vi "AutoMapper.vi"(8 "error in (no error)":errorcluster) -> (0 "error out 4":errorcluster={"status"=TRUE, "code"=1055, "source"="Property Node (arg 1) in AutoMapper.vi->Main.vi"})   [LabVIEW 2014]
uses:
  Libraries/Map Data Folder/All-Lines.ctl
  Libraries/Map Data Folder/LineCluster.ctl
  Libraries/Map Data Folder/LineConnection.ctl
  <vilib>/Utility/miscctls.llb/LVCursorListTypeDef.ctl
  <vilib>/Utility/miscctls.llb/LVRangeTypeDef.ctl
  <vilib>/Utility/miscctls.llb/LVPoint32TypeDef.ctl
  Controls/SwitchOp.ctl
  SwitchControl/Controls/ManualOveride.ctl
  SwitchControl/Controls/ManualState.ctl
  Libraries/Map Data Folder/Map Data.lvlib
  Libraries/Contact Data/Contact Data.lvlib
panel:
  in  "SwitchOp":T1[](array[typedef])
  out "Cursor List":T4
  out "output array":T5
  out "AutoMapper":cluster{cluster{"X":dbl, "Z":dbl}[]}[](graph)=[{[{"X"=1846.876, "Z"=5458.5}, {"X"=1845.414, "Z"=5458.5}, {"X"=1843.46, "Z"=5458.5}, {"X"=1841.231, "Z"=5458.5}, {"X"=1838.753, "Z"=5458.5}, {"X"=1836.154, "Z"=5458.5}, {"X"=1833.319, "Z"=5458.5}, {"X"=1830.276, "Z"=5458.5}, {"X"=1827.045, "Z"=5458.5}, {"X"=1823.657, "Z"=5458.5}, {"X"=1820.23, "Z"=5458.5}, {"X"=1816.783, "Z"=5458.5}, {"X"=1813.318, "Z"=5458.5}, {"X"=1809.835, "Z"=5458.5}, {"X"=1806.336, "Z"=5458.5}, {"X"=1802.822, "Z"=5458.5}, {"X"=1799.293, "Z"=5458.5}, {"X"=1795.751, "Z"=5458.5}, {"X"=1792.197, "Z"=5458.5}, {"X"=1788.356, "Z"=5458.5}, {"X"=1784.777, "Z"=5458.5}, {"X"=1782.771, "Z"=5458.749}, {"X"=1781.189, "Z"=5458.5}, {"X"=1777.591, "Z"=5458.5}, {"X"=1775.817, "Z"=5458.5}, {"X"=1773.983, "Z"=5458.5}, {"X"=1772.669, "Z"=5458.5}, {"X"=1770.367, "Z"=5458.5}, {"X"=1769.342, "Z"=5458.5}, {"X"=1766.743, "Z"=5458.5}, {"X"=1763.943, "Z"=5458.5}, {"X"=1762.831, "Z"=5458.5}, {"X"=1759.192, "Z"=5458.5}, {"X"=1755.545, "Z"=5458.5}, {"X"=1751.893, "Z"=5458.5}, {"X"=1749.392, "Z"=5458.5}, {"X"=1748.234, "Z"=5458.5}, {"X"=1744.57, "Z"=5458.5}, {"X"=1743.098, "Z"=5458.5}, {"X"=1740.9, "Z"=5458.5}, {"X"=1737.225, "Z"=5458.5}, {"X"=1735.038, "Z"=5458.5}, {"X"=1733.546, "Z"=5458.5}, {"X"=1729.862, "Z"=5458.5}, {"X"=1726.174, "Z"=5458.5}, {"X"=1722.481, "Z"=5458.5}, {"X"=1718.785, "Z"=5458.507}, {"X"=1714.804, "Z"=5458.598}, {"X"=1711.11, "Z"=5458.842}, {"X"=1707.431, "Z"=5459.274}, {"X"=1703.781, "Z"=5459.918}, {"X"=1700.177, "Z"=5460.798}, {"X"=1696.639, "Z"=5461.934}, {"X"=1693.093, "Z"=5463.377}, {"X"=1689.52, "Z"=5465.176}, {"X"=1685.962, "Z"=5467.324}, {"X"=1682.433, "Z"=5469.784}, {"X"=1678.913, "Z"=5472.481}, {"X"=1675.343, "Z"=5475.315}, {"X"=1671.345, "Z"=5478.377}, {"X"=1667.401, "Z"=5481.085}, {"X"=1663.17, "Z"=5483.523}, {"X"=1658.281, "Z"=5485.722}, {"X"=1653.463, "Z"=5487.302}, {"X"=1648.432, "Z"=5488.426}, {"X"=1643.243, "Z"=5489.125}, {"X"=1637.941, "Z"=5489.446}, {"X"=1632.556, "Z"=5489.5}, {"X"=1627.102, "Z"=5489.5}, {"X"=1621.583, "Z"=5489.5}, {"X"=1615.139, "Z"=5489.5}, {"X"=1609.49, "Z"=5489.5}, {"X"=1603.785, "Z"=5489.5}, {"X"=1598.026, "Z"=5489.5}, {"X"=1591.766, "Z"=5489.5}, {"X"=1585.902, "Z"=5489.5}, {"X"=1579.991, "Z"=5489.5}, {"X"=1573.574, "Z"=5489.5}, {"X"=1567.106, "Z"=5489.5}, {"X"=1561.057, "Z"=5489.5}, {"X"=1554.968, "Z"=5489.5}, {"X"=1548.839, "Z"=5489.5}, {"X"=1542.673, "Z"=5489.5}, {"X"=1536.471, "Z"=5489.5}, {"X"=1530.234, "Z"=5489.5}, {"X"=1523.963, "Z"=5489.5}, {"X"=1517.66, "Z"=5489.5}, {"X"=1511.326, "Z"=5489.5}, {"X"=1504.961, "Z"=5489.5}, {"X"=1498.073, "Z"=5489.5}, {"X"=1491.648, "Z"=5489.5}, {"X"=1485.196, "Z"=5489.5}, {"X"=1478.717, "Z"=5489.5}, {"X"=1472.213, "Z"=5489.5}, {"X"=1465.683, "Z"=5489.502}, {"X"=1458.638, "Z"=5489.822}, {"X"=1452.145, "Z"=5490.832}, {"X"=1445.783, "Z"=5492.571}, {"X"=1439.639, "Z"=5495.023}, {"X"=1433.355, "Z"=5498.431}, {"X"=1427.912, "Z"=5502.268}, {"X"=1422.92, "Z"=5506.705}, {"X"=1418.125, "Z"=5512.094}, {"X"=1414.278, "Z"=5517.602}, {"X"=1411.074, "Z"=5523.528}, {"X"=1408.565, "Z"=5529.8}, {"X"=1406.792, "Z"=5536.335}, {"X"=1405.782, "Z"=5543.048}, {"X"=1405.501, "Z"=5549.849}, {"X"=1405.5, "Z"=5556.676}, {"X"=1405.5, "Z"=5563.519}, {"X"=1405.5, "Z"=5570.376}, {"X"=1405.5, "Z"=5577.248}, {"X"=1405.5, "Z"=5584.126}, {"X"=1405.5, "Z"=5590.852}, {"X"=1405.5, "Z"=5597.365}, {"X"=1405.5, "Z"=5604.141}, {"X"=1405.5, "Z"=5610.209}, {"X"=1405.5, "Z"=5616.063}, {"X"=1405.5, "Z"=5621.699}, {"X"=1405.5, "Z"=5627.118}, {"X"=1405.5, "Z"=5631.758}, {"X"=1405.5, "Z"=5634.602}]}, {[{"X"=1401.5, "Z"=5594.986}, {"X"=1401.5, "Z"=5593.692}, {"X"=1401.5, "Z"=5586.908}, {"X"=1401.5, "Z"=5585.809}, {"X"=1401.5, "Z"=5584.365}, {"X"=1401.5, "Z"=5582.58}, {"X"=1401.5, "Z"=5580.516}, {"X"=1401.5, "Z"=5578.212}, {"X"=1401.5, "Z"=5575.693}, {"X"=1401.5, "Z"=5572.979}, {"X"=1401.5, "Z"=5570.085}, {"X"=1401.5, "Z"=5567.024}, {"X"=1401.5, "Z"=5563.807}, {"X"=1401.5, "Z"=5560.442}, {"X"=1401.5, "Z"=5556.938}, {"X"=1401.5, "Z"=5553.299}, {"X"=1401.5, "Z"=5549.534}, {"X"=1401.502, "Z"=5545.646}, {"X"=1401.6, "Z"=5541.644}, {"X"=1401.939, "Z"=5537.543}, {"X"=1402.583, "Z"=5533.368}, {"X"=1403.554, "Z"=5529.149}, {"X"=1404.983, "Z"=5524.592}, {"X"=1406.681, "Z"=5520.384}, {"X"=1408.745, "Z"=5516.235}, {"X"=1411.382, "Z"=5511.877}, {"X"=1414.218, "Z"=5507.974}, {"X"=1417.682, "Z"=5503.971}, {"X"=1421.274, "Z"=5500.485}, {"X"=1425.214, "Z"=5497.263}, {"X"=1429.827, "Z"=5494.138}, {"X"=1434.432, "Z"=5491.6}, {"X"=1439.704, "Z"=5489.309}, {"X"=1444.857, "Z"=5487.633}, {"X"=1450.636, "Z"=5486.355}, {"X"=1457.03, "Z"=5485.632}, {"X"=1462.687, "Z"=5485.499}, {"X"=1468.863, "Z"=5485.5}, {"X"=1474.669, "Z"=5485.5}, {"X"=1480.997, "Z"=5485.5}, {"X"=1486.943, "Z"=5485.5}, {"X"=1492.955, "Z"=5485.5}, {"X"=1499.501, "Z"=5485.5}, {"X"=1505.645, "Z"=5485.5}, {"X"=1512.332, "Z"=5485.5}, {"X"=1518.605, "Z"=5485.5}, {"X"=1524.939, "Z"=5485.5}, {"X"=1531.332, "Z"=5485.5}, {"X"=1537.784, "Z"=5485.5}, {"X"=1544.796, "Z"=5485.5}, {"X"=1551.367, "Z"=5485.5}, {"X"=1557.995, "Z"=5485.5}, {"X"=1564.677, "Z"=5485.5}, {"X"=1571.415, "Z"=5485.5}, {"X"=1578.206, "Z"=5485.5}, {"X"=1585.051, "Z"=5485.5}, {"X"=1591.948, "Z"=5485.5}, {"X"=1599.434, "Z"=5485.5}, {"X"=1606.438, "Z"=5485.5}, {"X"=1613.494, "Z"=5485.5}, {"X"=1620.599, "Z"=5485.5}, {"X"=1627.753, "Z"=5485.5}, {"X"=1634.956, "Z"=5485.444}, {"X"=1642.182, "Z"=5484.911}, {"X"=1649.898, "Z"=5483.451}, {"X"=1656.845, "Z"=5481.087}, {"X"=1663.408, "Z"=5477.702}, {"X"=1669.536, "Z"=5473.49}, {"X"=1675.426, "Z"=5468.866}, {"X"=1680.506, "Z"=5465.006}, {"X"=1681.928, "Z"=5464.014}, {"X"=1683.425, "Z"=5463.025}, {"X"=1685.221, "Z"=5461.92}, {"X"=1686.784, "Z"=5461.032}, {"X"=1688.448, "Z"=5460.162}, {"X"=1689.514, "Z"=5459.645}, {"X"=1692.148, "Z"=5458.502}, {"X"=1694.602, "Z"=5457.596}, {"X"=1696.064, "Z"=5457.125}, {"X"=1697.726, "Z"=5456.647}, {"X"=1700.823, "Z"=5455.909}, {"X"=1703.533, "Z"=5455.412}, {"X"=1707.824, "Z"=5454.868}, {"X"=1711.202, "Z"=5454.627}, {"X"=1715.302, "Z"=5454.512}, {"X"=1718.959, "Z"=5454.5}, {"X"=1722.952, "Z"=5454.5}, {"X"=1726.761, "Z"=5454.5}, {"X"=1728.143, "Z"=5454.5}, {"X"=1729.73, "Z"=5454.5}, {"X"=1730.767, "Z"=5454.5}, {"X"=1734.605, "Z"=5454.5}, {"X"=1743.09, "Z"=5454.5}, {"X"=1744.603, "Z"=5454.5}, {"X"=1746.155, "Z"=5454.5}, {"X"=1747.277, "Z"=5454.5}, {"X"=1748.888, "Z"=5454.5}, {"X"=1750.944, "Z"=5454.5}, {"X"=1752.514, "Z"=5454.5}, {"X"=1754.254, "Z"=5454.5}, {"X"=1755.425, "Z"=5454.5}, {"X"=1756.626, "Z"=5454.5}, {"X"=1758.764, "Z"=5454.5}, {"X"=1760.384, "Z"=5454.5}, {"X"=1761.686, "Z"=5454.5}, {"X"=1763.01, "Z"=5454.5}, {"X"=1765.01, "Z"=5454.5}, {"X"=1766.549, "Z"=5454.5}, {"X"=1768.513, "Z"=5454.5}, {"X"=1769.936, "Z"=5454.5}, {"X"=1771.064, "Z"=5454.5}, {"X"=1772.836, "Z"=5454.5}, {"X"=1774.09, "Z"=5454.5}, {"X"=1775.959, "Z"=5454.5}, {"X"=1777.402, "Z"=5454.5}, {"X"=1779.54, "Z"=5454.5}, {"X"=1781.08, "Z"=5454.5}, {"X"=1783.115, "Z"=5454.5}, {"X"=1786.384, "Z"=5454.5}, {"X"=1788.654, "Z"=5454.5}, {"X"=1791.126, "Z"=5454.5}, {"X"=1794.012, "Z"=5454.5}, {"X"=1795.833, "Z"=5454.5}, {"X"=1799.183, "Z"=5454.5}, {"X"=1800.864, "Z"=5454.5}, {"X"=1804.158, "Z"=5454.5}, {"X"=1805.5, "Z"=5454.5}, {"X"=1808.926, "Z"=5454.5}, {"X"=1810.101, "Z"=5454.5}, {"X"=1813.478, "Z"=5454.5}, {"X"=1814.667, "Z"=5454.5}, {"X"=1817.8, "Z"=5454.5}, {"X"=1819.199, "Z"=5454.5}, {"X"=1821.878, "Z"=5454.5}, {"X"=1823.697, "Z"=5454.5}, {"X"=1825.693, "Z"=5454.5}, {"X"=1828.16, "Z"=5454.5}, {"X"=1829.224, "Z"=5454.5}, {"X"=1832.575, "Z"=5454.5}, {"X"=1835.51, "Z"=5454.5}, {"X"=1837.151, "Z"=5454.5}, {"X"=1840.345, "Z"=5454.5}]}, {[{"X"=1799.071, "Z"=5459.117}, {"X"=1801.212, "Z"=5460.627}, {"X"=1803.251, "Z"=5462.366}, {"X"=1805.161, "Z"=5464.328}, {"X"=1807.039, "Z"=5466.683}, {"X"=1808.583, "Z"=5469.081}, {"X"=1809.905, "Z"=5471.669}, {"X"=1810.976, "Z"=5474.425}, {"X"=1811.769, "Z"=5477.325}, {"X"=1812.261, "Z"=5480.341}, {"X"=1812.464, "Z"=5483.437}, {"X"=1812.5, "Z"=5486.593}, {"X"=1812.5, "Z"=5489.795}, {"X"=1812.5, "Z"=5493.04}, {"X"=1812.5, "Z"=5496.583}, {"X"=1812.5, "Z"=5499.916}, {"X"=1812.5, "Z"=5503.29}, {"X"=1812.5, "Z"=5506.969}, {"X"=1812.5, "Z"=5509.183}, {"X"=1812.5, "Z"=5510.425}, {"X"=1812.5, "Z"=5513.919}, {"X"=1812.5, "Z"=5517.45}, {"X"=1812.5, "Z"=5521.018}, {"X"=1812.5, "Z"=5524.901}, {"X"=1812.5, "Z"=5528.543}, {"X"=1812.5, "Z"=5530.174}, {"X"=1812.5, "Z"=5532.504}, {"X"=1812.5, "Z"=5536.217}, {"X"=1812.5, "Z"=5539.963}, {"X"=1812.5, "Z"=5544.034}, {"X"=1812.5, "Z"=5547.847}, {"X"=1812.5, "Z"=5551.692}, {"X"=1812.5, "Z"=5555.692}, {"X"=1812.5, "Z"=5559.942}, {"X"=1812.5, "Z"=5564.425}, {"X"=1812.5, "Z"=5569.129}, {"X"=1812.5, "Z"=5574.042}, {"X"=1812.5, "Z"=5579.155}, {"X"=1812.5, "Z"=5584.457}, {"X"=1812.5, "Z"=5589.942}, {"X"=1812.5, "Z"=5595.603}, {"X"=1812.5, "Z"=5601.432}, {"X"=1812.5, "Z"=5607.425}, {"X"=1812.5, "Z"=5613.577}, {"X"=1812.5, "Z"=5617.536}, {"X"=1812.5, "Z"=5619.882}, {"X"=1812.5, "Z"=5626.335}, {"X"=1812.5, "Z"=5633.447}, {"X"=1812.5, "Z"=5639.076}, {"X"=1812.5, "Z"=5640.722}, {"X"=1812.5, "Z"=5647.62}, {"X"=1812.5, "Z"=5654.65}, {"X"=1812.5, "Z"=5660.65}, {"X"=1812.5, "Z"=5661.812}, {"X"=1812.5, "Z"=5669.666}, {"X"=1812.5, "Z"=5677.089}, {"X"=1812.5, "Z"=5682.259}, {"X"=1812.5, "Z"=5684.634}, {"X"=1812.5, "Z"=5692.297}, {"X"=1812.5, "Z"=5700.065}, {"X"=1812.5, "Z"=5703.903}, {"X"=1812.5, "Z"=5707.786}, {"X"=1812.5, "Z"=5715.309}, {"X"=1812.5, "Z"=5722.623}, {"X"=1812.5, "Z"=5725.581}, {"X"=1812.5, "Z"=5729.728}, {"X"=1812.5, "Z"=5736.621}, {"X"=1812.5, "Z"=5743.341}, {"X"=1812.5, "Z"=5747.281}, {"X"=1812.5, "Z"=5750.016}, {"X"=1812.5, "Z"=5756.657}, {"X"=1812.474, "Z"=5763.262}, {"X"=1812.185, "Z"=5769.825}, {"X"=1811.458, "Z"=5776.319}, {"X"=1810.766, "Z"=5782.782}, {"X"=1810.518, "Z"=5789.243}, {"X"=1810.506, "Z"=5790.562}, {"X"=1810.5, "Z"=5795.676}, {"X"=1810.5, "Z"=5802.074}, {"X"=1810.5, "Z"=5808.438}, {"X"=1810.5, "Z"=5812.263}, {"X"=1810.5, "Z"=5814.768}, {"X"=1810.5, "Z"=5821.063}, {"X"=1810.5, "Z"=5827.804}, {"X"=1810.5, "Z"=5834.027}, {"X"=1810.5, "Z"=5835.615}, {"X"=1810.498, "Z"=5840.216}, {"X"=1810.209, "Z"=5846.832}, {"X"=1809.284, "Z"=5852.872}, {"X"=1808.217, "Z"=5857.088}, {"X"=1807.703, "Z"=5858.738}, {"X"=1805.493, "Z"=5864.361}, {"X"=1802.455, "Z"=5870.07}, {"X"=1799.074, "Z"=5874.99}, {"X"=1798.165, "Z"=5876.137}, {"X"=1795.206, "Z"=5879.491}, {"X"=1790.905, "Z"=5883.531}, {"X"=1786.226, "Z"=5887.07}, {"X"=1780.833, "Z"=5890.283}, {"X"=1775.559, "Z"=5892.685}, {"X"=1770.093, "Z"=5894.503}, {"X"=1764.5, "Z"=5895.731}, {"X"=1760.983, "Z"=5896.193}, {"X"=1758.844, "Z"=5896.365}, {"X"=1753.186, "Z"=5896.5}, {"X"=1747.553, "Z"=5896.5}, {"X"=1741.942, "Z"=5896.5}, {"X"=1739.313, "Z"=5896.5}, {"X"=1736.351, "Z"=5896.5}, {"X"=1730.782, "Z"=5896.5}, {"X"=1725.234, "Z"=5896.5}, {"X"=1719.705, "Z"=5896.5}, {"X"=1717.619, "Z"=5896.5}, {"X"=1714.169, "Z"=5896.5}, {"X"=1708.622, "Z"=5896.5}, {"X"=1703.065, "Z"=5896.5}, {"X"=1697.496, "Z"=5896.5}, {"X"=1695.925, "Z"=5896.5}, {"X"=1691.917, "Z"=5896.5}, {"X"=1686.327, "Z"=5896.5}, {"X"=1680.726, "Z"=5896.5}, {"X"=1675.115, "Z"=5896.5}, {"X"=1672.569, "Z"=5896.5}, {"X"=1669.494, "Z"=5896.5}, {"X"=1663.862, "Z"=5896.5}, {"X"=1658.219, "Z"=5896.5}, {"X"=1652.567, "Z"=5896.5}, {"X"=1650.865, "Z"=5896.5}, {"X"=1646.905, "Z"=5896.5}, {"X"=1641.232, "Z"=5896.5}, {"X"=1635.55, "Z"=5896.5}, {"X"=1629.857, "Z"=5896.5}, {"X"=1624.155, "Z"=5896.5}, {"X"=1618.443, "Z"=5896.5}, {"X"=1612.723, "Z"=5896.431}, {"X"=1607.023, "Z"=5895.916}, {"X"=1601.407, "Z"=5894.762}, {"X"=1595.949, "Z"=5892.975}, {"X"=1590.721, "Z"=5890.578}, {"X"=1587.306, "Z"=5888.597}, {"X"=1585.788, "Z"=5887.6}, {"X"=1581.215, "Z"=5884.081}, {"X"=1577.061, "Z"=5880.062}, {"X"=1573.379, "Z"=5875.595}, {"X"=1571.948, "Z"=5873.537}, {"X"=1570.222, "Z"=5870.733}, {"X"=1567.633, "Z"=5865.535}, {"X"=1565.653, "Z"=5860.067}, {"X"=1564.313, "Z"=5854.399}, {"X"=1563.604, "Z"=5848.158}, {"X"=1563.5, "Z"=5842.311}, {"X"=1563.5, "Z"=5836.453}, {"X"=1563.5, "Z"=5831.83}, {"X"=1563.503, "Z"=5830.586}, {"X"=1563.759, "Z"=5824.72}, {"X"=1564.64, "Z"=5818.91}, {"X"=1566.193, "Z"=5813.234}, {"X"=1567.159, "Z"=5810.611}, {"X"=1568.396, "Z"=5807.769}, {"X"=1571.222, "Z"=5802.589}, {"X"=1574.634, "Z"=5797.764}, {"X"=1578.584, "Z"=5793.357}, {"X"=1583.02, "Z"=5789.43}, {"X"=1587.888, "Z"=5786.037}, {"X"=1593.125, "Z"=5783.229}, {"X"=1597.481, "Z"=5781.454}, {"X"=1598.66, "Z"=5781.05}, {"X"=1604.421, "Z"=5779.535}, {"X"=1610.328, "Z"=5778.705}, {"X"=1616.762, "Z"=5778.499}, {"X"=1618.836, "Z"=5778.5}, {"X"=1622.75, "Z"=5778.5}, {"X"=1628.747, "Z"=5778.5}, {"X"=1635.212, "Z"=5778.5}, {"X"=1641.224, "Z"=5778.5}, {"X"=1647.244, "Z"=5778.5}, {"X"=1653.27, "Z"=5778.5}, {"X"=1659.304, "Z"=5778.5}, {"X"=1662.216, "Z"=5778.5}, {"X"=1665.346, "Z"=5778.5}, {"X"=1671.394, "Z"=5778.5}, {"X"=1677.45, "Z"=5778.5}, {"X"=1683.513, "Z"=5778.5}, {"X"=1689.583, "Z"=5778.5}, {"X"=1695.66, "Z"=5778.5}, {"X"=1701.744, "Z"=5778.5}, {"X"=1705.597, "Z"=5778.5}, {"X"=1707.835, "Z"=5778.5}, {"X"=1713.932, "Z"=5778.533}, {"X"=1720.03, "Z"=5778.8}, {"X"=1726.102, "Z"=5779.467}, {"X"=1728.88, "Z"=5779.922}, {"X"=1732.127, "Z"=5780.524}, {"X"=1738.16, "Z"=5781.57}, {"X"=1744.255, "Z"=5782.219}, {"X"=1750.386, "Z"=5782.471}, {"X"=1756.53, "Z"=5782.458}, {"X"=1762.675, "Z"=5782.2}, {"X"=1768.804, "Z"=5781.616}, {"X"=1771.5, "Z"=5781.231}, {"X"=1774.883, "Z"=5780.617}, {"X"=1781.307, "Z"=5778.941}, {"X"=1787.045, "Z"=5776.677}, {"X"=1792.387, "Z"=5773.591}, {"X"=1797.105, "Z"=5769.613}, {"X"=1800.993, "Z"=5764.814}, {"X"=1803.959, "Z"=5759.385}, {"X"=1806.054, "Z"=5753.552}, {"X"=1807.41, "Z"=5747.494}, {"X"=1808.212, "Z"=5740.847}, {"X"=1808.478, "Z"=5734.627}, {"X"=1808.5, "Z"=5728.394}, {"X"=1808.5, "Z"=5722.154}, {"X"=1808.5, "Z"=5715.908}, {"X"=1808.5, "Z"=5709.657}, {"X"=1808.5, "Z"=5703.4}, {"X"=1808.5, "Z"=5702.389}, {"X"=1808.5, "Z"=5697.137}, {"X"=1808.5, "Z"=5695.208}, {"X"=1808.5, "Z"=5688.938}, {"X"=1808.5, "Z"=5684.571}, {"X"=1808.5, "Z"=5682.661}, {"X"=1808.5, "Z"=5676.379}, {"X"=1808.5, "Z"=5670.091}, {"X"=1808.5, "Z"=5667.105}, {"X"=1808.5, "Z"=5663.798}, {"X"=1808.5, "Z"=5657.499}, {"X"=1808.5, "Z"=5650.709}, {"X"=1808.5, "Z"=5644.399}, {"X"=1808.5, "Z"=5638.083}, {"X"=1808.5, "Z"=5633.261}, {"X"=1808.5, "Z"=5631.762}, {"X"=1808.5, "Z"=5625.435}, {"X"=1808.5, "Z"=5618.616}, {"X"=1808.5, "Z"=5616.902}, {"X"=1808.5, "Z"=5612.278}, {"X"=1808.5, "Z"=5605.935}, {"X"=1808.5, "Z"=5600.93}, {"X"=1808.5, "Z"=5599.586}, {"X"=1808.5, "Z"=5593.233}, {"X"=1808.5, "Z"=5586.874}, {"X"=1808.5, "Z"=5585.356}, {"X"=1808.5, "Z"=5580.51}, {"X"=1808.5, "Z"=5574.141}, {"X"=1808.5, "Z"=5570.192}, {"X"=1808.5, "Z"=5567.766}, {"X"=1808.5, "Z"=5561.387}, {"X"=1808.5, "Z"=5554.511}, {"X"=1808.5, "Z"=5548.122}, {"X"=1808.5, "Z"=5541.727}, {"X"=1808.5, "Z"=5535.327}, {"X"=1808.5, "Z"=5528.923}, {"X"=1808.5, "Z"=5527.287}, {"X"=1808.5, "Z"=5522.513}, {"X"=1808.5, "Z"=5516.099}, {"X"=1808.5, "Z"=5513.897}, {"X"=1808.5, "Z"=5509.68}, {"X"=1808.5, "Z"=5503.256}, {"X"=1808.5, "Z"=5500.992}, {"X"=1808.5, "Z"=5496.827}, {"X"=1808.5, "Z"=5490.394}, {"X"=1808.493, "Z"=5488.593}, {"X"=1808.223, "Z"=5483.969}, {"X"=1806.742, "Z"=5477.73}, {"X"=1803.914, "Z"=5471.969}, {"X"=1799.882, "Z"=5466.969}, {"X"=1794.848, "Z"=5462.971}, {"X"=1789.05, "Z"=5460.182}, {"X"=1791.793, "Z"=5461.305}]}]
  in  "Read file":bool
  in  "Save File":bool
  in  "Fullscale":bool
  out "NewRange":T8={"Minimum"=5741.677215189875, "Maximum"=5401.677215189877, "Increment"=20.0, "Minor Increment"=5.0, "Start"=5420.0}
  out "Active Tool":i32=1
  out "error out 3":errorcluster
  out "Coords 2":T9={"Horizontal"=1470, "Vertical"=503}
  in  "Force Switch":bool
  in  "Get switches":bool
  out "Range":T10={"XScale.Maximum"=5216.950181278341, "XScale.Minimum"=5216.6897529125745, "YScale.Maximum"=7077.235845221711, "YScale.Minimum"=7074.783170378638}
  out "Delete zoom":bool
  in  "Any point?":bool=TRUE
  in  "Split Line":bool
  in  "Zoom\ndelete":bool
  in  "Display wait":u32=2000
  out "Dwell":u32=199
  in  "Single train?":bool
  in  "Clear Cursors":bool
  in  "Update switches":bool
  in  "Delete index":i32
  in  "Delete Array":bool
  out "Array size":i32=3
  in  "Clear?":bool
  out "Nearest Line":i32
  in  "Min diff":dbl=1.0
  in  "Train index":i32=1
  out "New array":bool
  out "Deleted":bool=TRUE
  in  "Pause":bool
  in  "milliseconds to wait":u32=200
  in  "Save Map":bool
  in  "Load Cursors":bool
  in  "Add inbetween":bool
  in  "Delete selected":bool
  in  "Save Cursors":bool
  in  "Delete Station":bool
  in  "Name":string="Station"
  in  "Add Station":bool
  in  "Load Maps":bool
  in  "stop":bool=TRUE
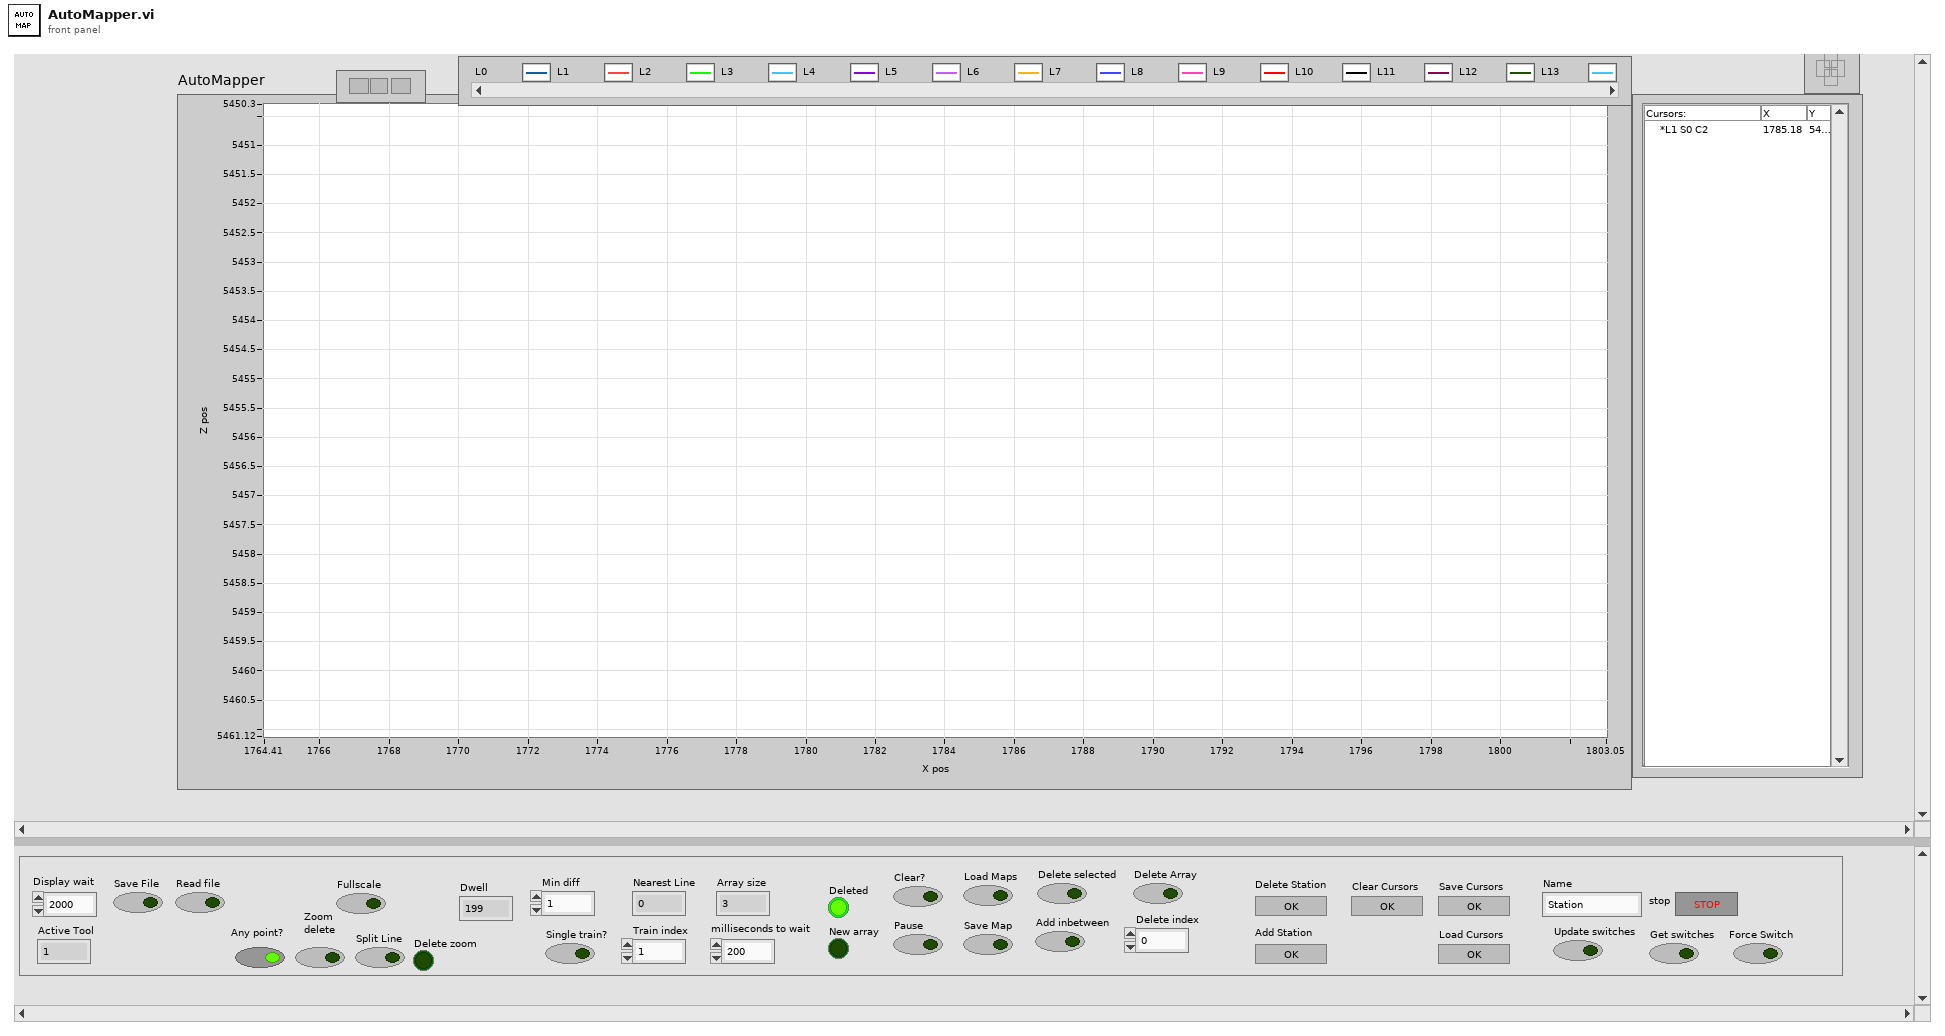
[diagram p1: front panel]
types:
  T1 = typedef "SwitchOp.ctl" = cluster{"Switch operational":bool, "Switch State":bool, "Manual Overide":T2, "Manual State":T3, "Switch\nPosition":cluster{"X":dbl, "Y":dbl, "Z":dbl}, "Index":i32, "Connection Index":i32, "Switch Index":i32, string}
  T2 = typedef "ManualOveride.ctl" = bool
  T3 = typedef "ManualState.ctl" = bool
  T4 = typedef "LVCursorListTypeDef.ctl" = cluster{"Name":string, "Color":u32, "Style":u8, "Point Style":u8, "Name Visible":bool, "Allow Drag":bool, "Cursor Mode":u32, "Plot":i32, "Index":i32, "Position":cluster{"X":dbl, "Y":dbl}, "X Scale":u32, "Y Scale":u32, "Watch Plots":i32[], "Watch All Plots":bool, "Plot Area":i32, "Label Offset":cluster{"X":dbl, "Y":dbl}}[]
  T5 = typedef "Map Data.lvlib/All-Lines.ctl" = T6[]
  T6 = typedef "Map Data.lvlib/LineCluster.ctl" = cluster{"Line name":string, "Line array":cluster{"X":dbl, "Y":dbl, "Z":dbl}[], "Line connections":T7[]}
  T7 = typedef "Map Data.lvlib/LineConnection.ctl" = cluster{"Index":i32, "Switch Pos":cluster{"X":dbl, "Y":dbl, "Z":dbl}, "Switch operational":bool, "Switch State":bool, "Connection Index":i32, "Connection Pos":cluster{"X":dbl, "Y":dbl, "Z":dbl}, "LinePos Index":i32, "ConnectPos Index":i32, "Same direction?":bool, "Manual Overide":bool, "Manual State":bool}
  T8 = typedef "LVRangeTypeDef.ctl" = cluster{"Minimum":dbl, "Maximum":dbl, "Increment":dbl, "Minor Increment":dbl, "Start":dbl}
  T9 = typedef "LVPoint32TypeDef.ctl" = cluster{"Horizontal":i32, "Vertical":i32}
  T10 = cluster{"XScale.Maximum":dbl, "XScale.Minimum":dbl, "YScale.Maximum":dbl, "YScale.Minimum":dbl}
  T11 = cluster{"Line name":string, "Line array":cluster{"X":dbl, "Y":dbl, "Z":dbl}[], "Line connections":cluster{"Index":i32, "Switch Pos":cluster{"X":dbl, "Y":dbl, "Z":dbl}, "Switch operational":bool, "Switch State":bool, "Connection Index":i32, "Connection Pos":cluster{"X":dbl, "Y":dbl, "Z":dbl}, "LinePos Index":i32, "ConnectPos Index":i32, "Same direction?":bool}[]}[]
  T12 = enum32{"Invalid", "Standard", "Closed", "Hidden", "Minimized", "Maximized"}
  T13 = enum16{"Initialise", "Close", "Read", "Write", "Ask for File", ""}
  T14 = typedef "Contact Data.lvlib/Contact.ctl" = cluster{"ID":u32, "UUID":string, "Name":string, "Iteration":i32, "Posit Array":T15[], "Controls":T16, "DestArray":T17[], "SetSpeed":dbl, "Speed":dbl, "PathData":T19}
  T15 = typedef "Contact Data.lvlib/Position.ctl" = cluster{"X":dbl, "Y":dbl, "Z":dbl}
  T16 = typedef "Contact Data.lvlib/Controls.ctl" = cluster{"throttle":dbl, "brake":dbl, "horn":dbl, "wait":dbl}
  T17 = typedef "Contact Data.lvlib/DestinationCluster.ctl" = cluster{"Desination":string, "DestControls":T18, "Timer":u32, "Set Timer":u32, "Time Stamp":timestamp, "Repeat?":bool, "Optional Data":string, "Distance":dbl}
  T18 = typedef "Contact Data.lvlib/DesinationControls.ctl" = enum16{"Tracker", "Manual", "Stop", "Station DateTime", "Station Timer", "Maintain"}
  T19 = typedef "Contact Data.lvlib/PathData.ctl" = cluster{"Path Found?":bool, "Same Line +Dir?":bool, "Path":T20[]}
  T20 = typedef "ShortestPath.ctl" = cluster{"Line Index":i32, "Line Pos Index ":i32, "Prev Index ":i32, "Prev Pos Index":i32, "Distance":dbl}
  T21 = cluster{"Name":string, "Color":u32, "Style":u8, "Point Style":u8, "Name Visible":bool, "Allow Drag":bool, "Cursor Mode":u32, "Plot":i32, "Index":i32, "Position":cluster{"X":dbl, "Y":dbl}, "X Scale":u32, "Y Scale":u32, "Watch Plots":i32[], "Watch All Plots":bool, "Plot Area":i32, "Label Offset":cluster{"X":dbl, "Y":dbl}}
  T22 = cluster{"Shift":bool, "Ctrl":bool, "Alt":bool, "Cmd":bool, "Opt":bool}
  T23 = typedef "Map Data.lvlib/CursorList.ctl" = cluster{"Name":string, "Color":u32, "Style":u8, "Point Style":u8, "Name Visible":bool, "Allow Drag":bool, "Cursor Mode":u32, "Plot":i32, "Index":i32, "Position":cluster{"X":dbl, "Y":dbl}, "X Scale":u32, "Y Scale":u32, "Watch Plots":i32[], "Watch All Plots":bool, "Plot Area":i32, "Label Offset":cluster{"X":dbl, "Y":dbl}}[]
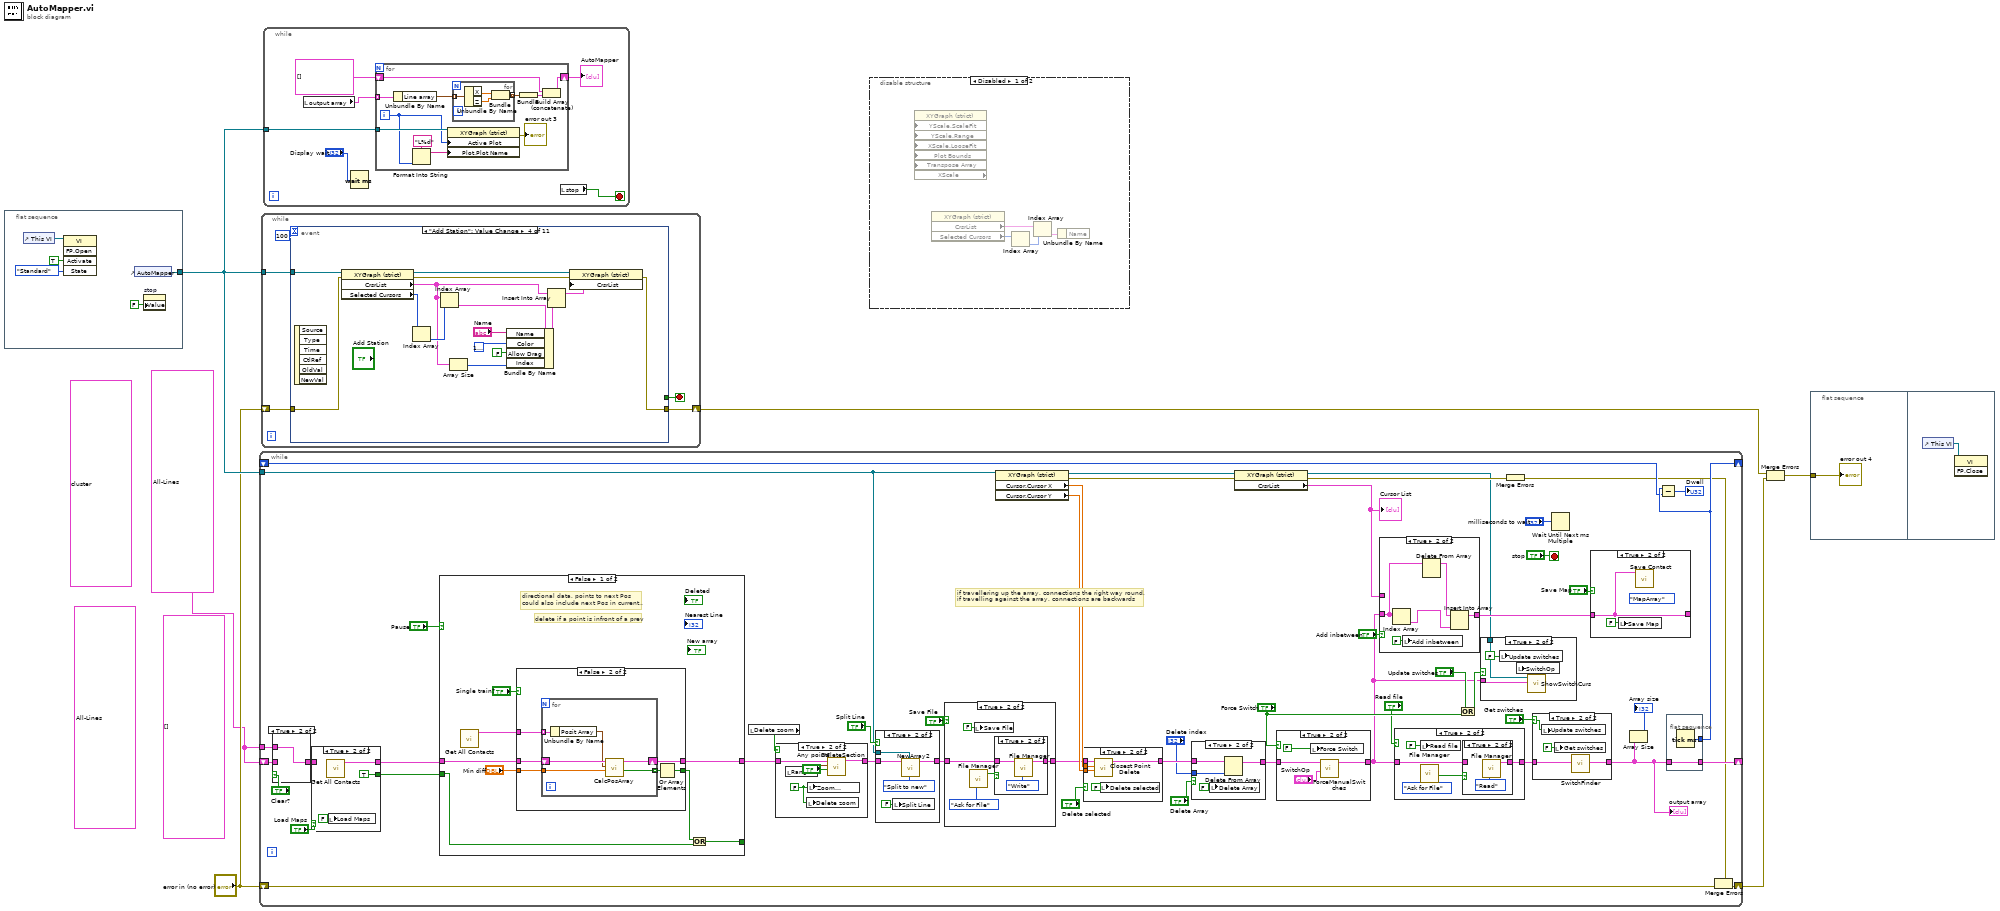
[diagram p0: block diagram]
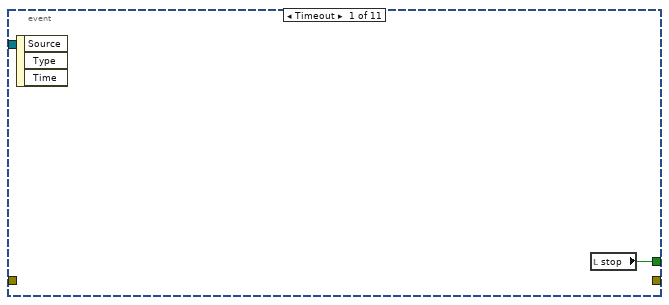
[diagram p3: hidden frame]
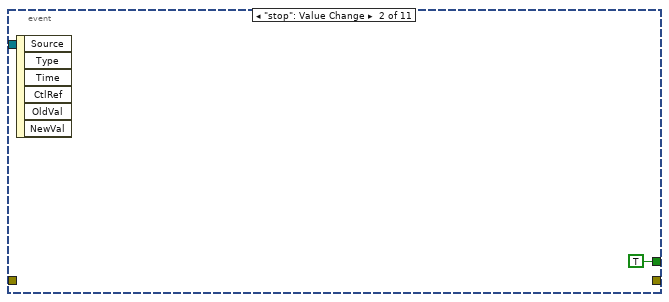
[diagram p4: hidden frame]
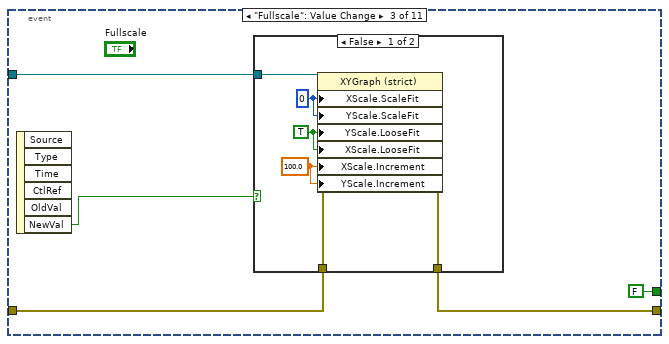
[diagram p5: hidden frame]
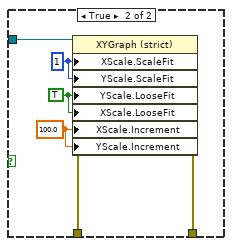
[diagram p6: hidden frame]
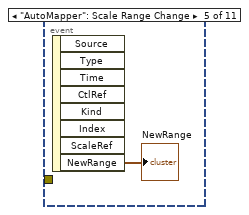
[diagram p7: hidden frame]
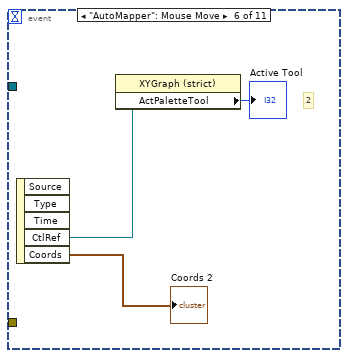
[diagram p8: hidden frame]
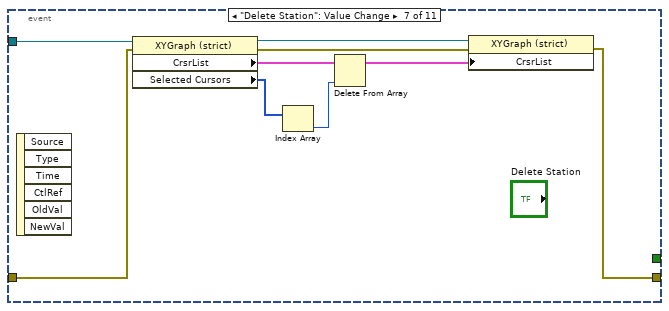
[diagram p9: hidden frame]
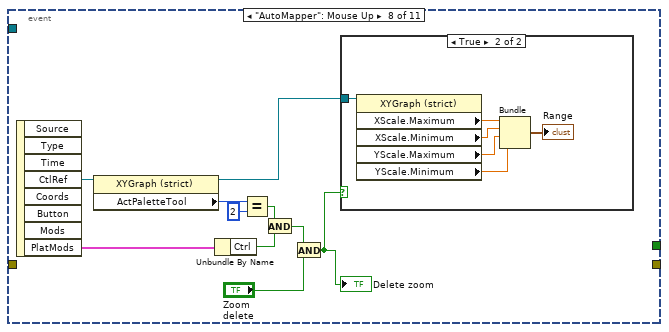
[diagram p10: hidden frame]
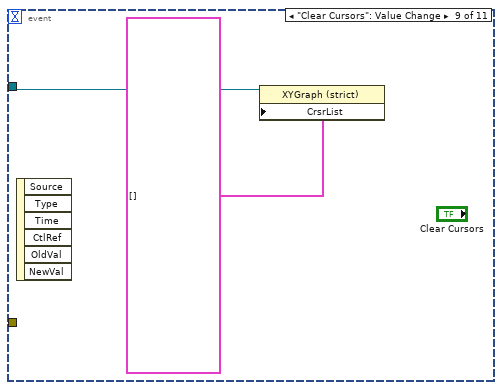
[diagram p12: hidden frame]
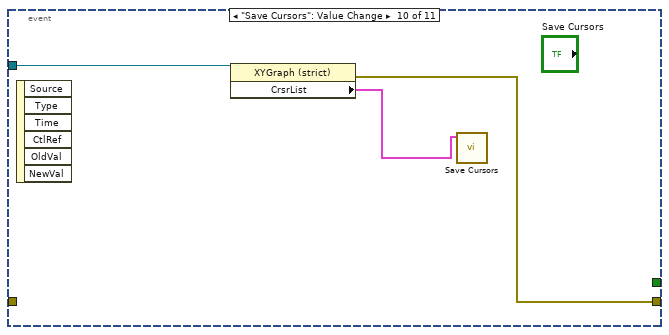
[diagram p13: hidden frame]
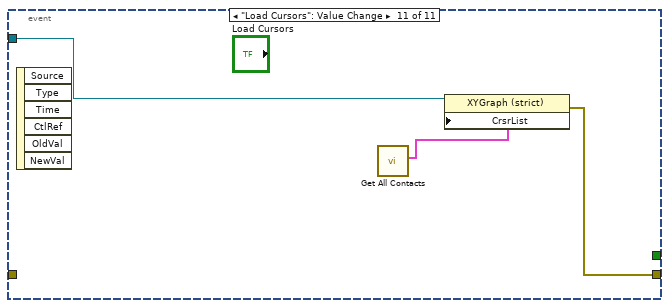
[diagram p14: hidden frame]
diagram:
  w1 = T5 data[18046B] ("output array")
  (unwired) T11 data[395744B] ("output array")
  (unwired) T5 data[395818B] ("output array")
  (unwired) T5 [] ("All Lines out")
  n1 = flat-sequence {
    tunnel: [w11] -> w4
    frame #0 {
      n2 = control-ref of="This VI"() -> (w9:refnum<vi>)
      n3 = invoke class="VI" method="FP.Open"(reference=w9, "Activate"=TRUE ("Activate?"), "State"=T12."Standard") -> ()  [unwired: 2 in, 5 out]
      n4 = control-ref of="AutoMapper"() -> (w11:refnum<vi>)
      n5 = property on="stop" class="Bool (strict)"("Value"=FALSE ("stop")) -> ()  [unwired: 2 in, 2 out]
    }
  }
  n6 = while {
    shift-right: [w26] -> _
    shift-left: w1 -> [w49]
    tunnel: w4 -> [w31]
    tunnel: w1 -> [w48]
    shift-right: [w35] -> _
    shift-left: _ -> [w34]
    shift-right: [w20] -> w3
    shift-left: "error in (no error)" -> [w18]
    stop <- "stop" stop-if-true
    # "if travellering up the array, connections the right way round, \nif travelling against the array, connections are backwards"
    n7 = case shown="True" "Clear?" {
      tunnel: w49 -> [w113 _]
      tunnel: [w113 w114] -> w39
      tunnel: w48 -> [_ w114]
      frame False {
      }
      frame True {
      }
    }
    n8 = case shown="True" "Load Maps" {
      tunnel: w39 -> [w160 _]
      tunnel: [w160 w162] -> w38
      tunnel: [FALSE TRUE] -> w37
      frame False {
      }
      frame True {
        n9 = call "Get All Contacts.vi"() -> ("All Lines out"=w162:T5)  [unwired: 9 in, 2 out]
        n10 = local write "Load Maps"(FALSE ("Boolean")) -> ()
      }
    }
    n11 = case shown="False" "Pause" {
      tunnel: [w120 w144] -> w28
      tunnel: w38 -> [w121 w144]
      tunnel: w37 -> [w115 w143]
      tunnel: [w116 w143] -> _
      frame False {
        # "delete if a point is infront of a prev"
        # "directional data, points to next Pos\ncould also include next Pos in current.."
        n12 = call "Get All Contacts.vi"() -> ("Contacts"=w122:T14[])  [unwired: 10 in, 1 out]
        n13 = case shown="False" "Single train?" {
          tunnel: w122 -> [w129 w133]
          tunnel: w121 -> [w128 w136]
          tunnel: [w127 w135] -> w120
          tunnel: "Min diff" -> [w126 w134]
          tunnel: [w123 w131] -> w117
          frame True {
            n14 = Index Array(array=w129, index="Train index") -> (element=w125:T14)
            n15 = Unbundle By Name(w125) -> ("Posit Array"=w124:T15[])
            n16 = call "CalcPosArray.vi"("Min diff"=w126, "Posit Array"=w124, "All Lines"=w128) -> ("Modified?"=w123:bool, "All Lines out"=w127:T5)  [unwired: 6 in, 1 out]
          }
          frame False {
            n17 = for {
              tunnel: w134 -> [w140]
              shift-right: [w141] -> w135
              shift-left: w136 -> [w142]
              tunnel: w133 -> [w138] mode=indexing
              tunnel: [w137] -> w132 mode=indexing
              n18 = Unbundle By Name(w138) -> ("Posit Array"=w139:T15[])
              n19 = call "CalcPosArray.vi"("Min diff"=w140, "Posit Array"=w139, "All Lines"=w142) -> ("Modified?"=w137:bool, "All Lines out"=w141:T5)  [unwired: 6 in, 1 out]
            }
            n20 = Or Array Elements(Boolean array=w132) -> (logical OR=w131:bool)
          }
        }
        n21 = Or(x=w117, y=w115) -> (x .or. y?=w116:bool)
      }
      frame True {
      }
    }
    n22 = local read "Delete zoom"() -> (w29:bool)
    n23 = case shown="True" w29 {
      tunnel: w28 -> [w90 w95]
      tunnel: [w90 w94] -> w30
      frame False {
      }
      frame True {
        w93 = FALSE ("Zoom delete")
        n24 = local read "Range"() -> (w92:T10)
        n25 = local write "Delete zoom"(w93) -> ()
        n26 = local write "Zoom\ndelete"(w93) -> ()
        n27 = call "DeleteSection.vi"("Any Point?"="Any point?", "Range"=w92, "All Lines"=w95) -> ("output array"=w94:T5)  [unwired: 7 in, 1 out]
      }
    }
    n28 = case shown="True" "Split Line" {
      tunnel: [w96 w99] -> w16
      tunnel: w30 -> [w96 w100]
      tunnel: w31 -> [_ w98]
      frame False {
      }
      frame True {
        n29 = local write "Split Line"(FALSE ("Split Line")) -> ()
        n30 = call "NewArray2.vi"("Function"=enum16{"Default", "Split to new"}."Split to new", "Map ref"=w98, "All Lines"=w100) -> ("output array"=w99:T5)  [unwired: 7 in, 1 out]
      }
    }
    n31 = case shown="True" "Save File" {
      tunnel: w16 -> [w70 w73]
      tunnel: [w70 w72] -> w15
      frame False {
      }
      frame True {
        n32 = call "File Manager.vi"("File Functions"=T13."Ask for File") -> ("cancelled"=w74:bool)  [unwired: 8 in, 2 out]
        n33 = local write "Save File"(FALSE ("Save File")) -> ()
        n34 = case shown="True" w74 {
          tunnel: w73 -> [w76 w79]
          tunnel: [w76 w78] -> w72
          frame False {
          }
          frame True {
            n35 = call "File Manager.vi"("File Functions"=T13."Write", "array in"=w79) -> ("array out"=w78:T5)  [unwired: 7 in, 2 out]
          }
        }
      }
    }
    n36 = property on="Property Node" class="XYGraph (strict)"(reference=w31) -> (reference out=w47:refnum<vi>, error out=w55:errorcluster, "Cursor.Cursor X"=w46:dbl, "Cursor.Cursor Y"=w45:dbl)  [unwired: 1 in]
    n37 = case shown="True" "Delete selected" {
      tunnel: w15 -> [w154 w157]
      tunnel: [w154 w158] -> w42
      tunnel: w46 -> [_ w156]
      tunnel: w45 -> [_ w155]
      frame False {
      }
      frame True {
        n38 = call "Closest Point Delete.vi"("Y in"=w155, "X in"=w156, "All Lines"=w157) -> ("output array"=w158:T5)  [unwired: 4 in, 4 out]
        n39 = local write "Delete selected"(FALSE ("Delete index")) -> ()
      }
    }
    n40 = case shown="True" "Delete Array" {
      tunnel: w42 -> [w108 w110]
      tunnel: [w108 w111] -> w24
      tunnel: "Delete index" -> [_ w109]
      frame False {
      }
      frame True {
        n41 = local write "Delete Array"(FALSE ("Add inbetween")) -> ()
        n42 = Delete From Array(array=w110, index=w109) -> (array with subset deleted=w111:T5)  [unwired: 1 in, 1 out]
      }
    }
    n43 = property on="Property Node" class="XYGraph (strict)"(reference=w47, error in=w55) -> (reference out=w33:refnum<vi>, error out=w54:errorcluster, "CrsrList"=w56:T4)
    "Cursor List" <- w56
    n44 = case shown="True" "Force Switch" {
      tunnel: [w80 w83] -> w13
      tunnel: w24 -> [w80 w84]
      frame False {
      }
      frame True {
        n45 = local write "Force Switch"(FALSE ("Manual \nswitch \nupdate")) -> ()
        n46 = call "ForceManualSwitches.vi"("Switch Op"="SwitchOp", "output array 2"=w84) -> ("output array 3"=w83:T5)  [unwired: 9 in]
      }
    }
    n47 = case shown="True" "Add inbetween" {
      tunnel: w13 -> [w148 w152]
      tunnel: w56 -> [_ _]
      tunnel: [w148 w150] -> w52
      frame False {
      }
      frame True {
        n48 = Index Array(array=w152) -> (element=w149:T6)  [unwired: 1 in]
        n49 = local write "Add inbetween"(FALSE ("Add inbetween")) -> ()
        n50 = Delete From Array(array=w152) -> (array with subset deleted=w151:T5)  [unwired: 2 in, 1 out]
        n51 = Insert Into Array(array=w151, new element=w149) -> (w150:T5)  [unwired: 1 in]
      }
    }
    n52 = case shown="True" "Read file" {
      tunnel: w13 -> [w61 w63]
      tunnel: [w61 w62] -> w12
      frame False {
      }
      frame True {
        n53 = call "File Manager.vi"("File Functions"=T13."Ask for File") -> ("cancelled"=w64:bool)  [unwired: 8 in, 2 out]
        n54 = local write "Read file"(FALSE ("Read file")) -> ()
        n55 = case shown="True" w64 {
          tunnel: w63 -> [w67 _]
          tunnel: [w67 w68] -> w62
          frame False {
          }
          frame True {
            n56 = call "File Manager.vi"("File Functions"=T13."Read") -> ("array out"=w68:T5)  [unwired: 8 in, 2 out]
          }
        }
      }
    }
    n57 = Or(x="Update switches", y="Force Switch") -> (x .or. y?=w22:bool)
    n58 = case shown="True" w22 {
      tunnel: w33 -> [_ w107]
      tunnel: w13 -> [_ w104]
      frame False {
      }
      frame True {
        n59 = local write "Update switches"(FALSE ("Update switches")) -> ()
        n60 = call "ShowSwitchCurs.vi"("All Lines"=w104, "Map"=w107) -> ("Switch Op"=w105:T1[])  [unwired: 8 in, 1 out]
        n61 = local write "SwitchOp"(w105) -> ()
      }
    }
    n62 = Merge Errors(w54) -> (w19:errorcluster)
    n63 = case shown="True" "Get switches" {
      selector: "Get switches" -> [_ w86]
      tunnel: [w85 w88] -> w25
      tunnel: w12 -> [w85 w89]
      frame False {
      }
      frame True {
        n64 = local write "Update switches"(w86) -> ()
        n65 = local write "Get switches"(FALSE ("Get switches")) -> ()
        n66 = call "SwitchFinder.vi"("All Lines in"=w89) -> ("All Lines out"=w88:T5)  [unwired: 10 in]
      }
    }
    "output array" <- w25
    n67 = Wait Until Next ms Multiple(millisecond multiple="milliseconds to wait") -> ()  [unwired: 1 out]
    n68 = case shown="True" "Save Map" {
      tunnel: [w145 w146] -> _
      tunnel: w52 -> [w145 w146]
      frame False {
      }
      frame True {
        (unwired) enum16{"MapArray", "Cursor"}."MapArray" ("Function")
        n69 = local write "Save Map"(FALSE ("Boolean")) -> ()
        n70 = call "Save Contact.vi"("All Lines"=w146) -> ()  [unwired: 9 in, 2 out]
      }
    }
    n71 = Array Size(array=w25) -> (size(s)=→"Array size":i32)
    n72 = Subtract(x=w35, y=w34) -> (x-y=→"Dwell":u32)
    n73 = flat-sequence {
      tunnel: w25 -> [w103]
      tunnel: [w103] -> w26
      tunnel: [w102] -> w35
      frame #0 {
        n74 = Tick Count (ms)() -> (millisecond timer value=w102:u32)
      }
    }
    n75 = Merge Errors(w19, w18) -> (w20:errorcluster)
  }
  n76 = while {
    tunnel: w4 -> [w168]
    shift-right: [w167] -> w6
    shift-left: "error in (no error)" -> [w166]
    stop <- w165 stop-if-true
    n77 = event shown="[3] \"Add Station\": Value Change" {
      selector: _ -> [_ _ _ _ _ _ _ _ _ _ _]
      dyn-events: _ -> [_ _ _ _ _ _ _ _ _ _ _]
      timeout: 100 -> [_ _ _ _ _ _ _ _ _ _ _]
      tunnel: [w170 TRUE ("stop") FALSE ("stop") _ _ _ _ _ _ _ _] -> w165
      tunnel: w168 -> [_ _ w172 w201 _ _ w216 _ w234 w237 w240]
      tunnel: [_ _ w174 w190 _ _ w208 _ _ w236 w239] -> w167
      tunnel: w166 -> [_ _ w175 w189 _ _ w210 _ _ _ _]
      event Timeout {
        n78 = event-data() -> ()  [unwired: 1 in, 3 out]
        n79 = local read "stop"() -> (w170:bool)
      }
      event "stop": Value Change {
        n80 = event-data() -> ()  [unwired: 1 in, 6 out]
      }
      event "Fullscale": Value Change {
        n81 = event-data() -> ("NewVal"=w173:bool)  [unwired: 1 in, 5 out]
        n82 = case shown="False" w173 {
          tunnel: w172 -> [w177 w186]
          tunnel: w175 -> [w178 w185]
          tunnel: [w179 w184] -> w174
          frame False {
            w180 = 100.0 ("X Scale.Range:Increment")
            w181 = TRUE ("Y Scale.Loose Fit")
            w182 = u8 0 ("X Scale.Scale Fit")
            n83 = property class="XYGraph (strict)"(reference=w177, error in=w178, "XScale.ScaleFit"=w182, "YScale.ScaleFit"=w182, "YScale.LooseFit"=w181, "XScale.LooseFit"=w181, "XScale.Increment"=w180, "YScale.Increment"=w180) -> (error out=w179:errorcluster)  [unwired: 1 out]
          }
          frame True {
            w183 = 100.0 ("X Scale.Range:Increment")
            w187 = TRUE ("Y Scale.Loose Fit")
            w188 = u8 1 ("X Scale.Scale Fit")
            n84 = property class="XYGraph (strict)"(reference=w186, error in=w185, "XScale.ScaleFit"=w188, "YScale.ScaleFit"=w188, "YScale.LooseFit"=w187, "XScale.LooseFit"=w187, "XScale.Increment"=w183, "YScale.Increment"=w183) -> (error out=w184:errorcluster)  [unwired: 1 out]
          }
        }
      }
      event "Add Station": Value Change {
        n85 = event-data() -> ()  [unwired: 1 in, 6 out]
        n86 = property on="Property Node" class="XYGraph (strict)"(reference=w201, error in=w189) -> (reference out=w200:refnum<vi>, error out=w191:errorcluster, "CrsrList"=w193:T4, "Selected Cursors"=w202:u32[])
        n87 = Index Array(array=w202) -> (element=w203:u32)  [unwired: 1 in]
        n88 = Index Array(array=w193, index=w203) -> (element=w198:T21)
        n89 = Array Size(array=w193) -> (size(s)=w192:i32)
        n90 = Bundle By Name(cluster=w198, "Name"="Name", "Color"=u32 16777222, "Allow Drag"=FALSE, "Index"=w192) -> (w197:T21)
        n91 = Insert Into Array(array=w193, new element=w197) -> (w199:T4)  [unwired: 1 in]
        n92 = property on="Property Node" class="XYGraph (strict)"(reference=w200, error in=w191, "CrsrList"=w199) -> (error out=w190:errorcluster)  [unwired: 1 out]
      }
      event "AutoMapper": Scale Range Change {
        n93 = event-data() -> ("NewRange"=→"NewRange":T8)  [unwired: 1 in, 7 out]
      }
      event "AutoMapper": Mouse Move {
        # "2"
        n94 = event-data() -> ("CtlRef"=w206:refnum<vi>, "Coords"=→"Coords 2":T9)  [unwired: 1 in, 3 out]
        n95 = property class="XYGraph (strict)"(reference=w206) -> ("ActPaletteTool"=→"Active Tool":i32)  [unwired: 1 in, 2 out]
      }
      event "Delete Station": Value Change {
        n96 = event-data() -> ()  [unwired: 1 in, 6 out]
        n97 = property on="Property Node" class="XYGraph (strict)"(reference=w216, error in=w210) -> (reference out=w214:refnum<vi>, error out=w209:errorcluster, "CrsrList"=w213:T4, "Selected Cursors"=w215:u32[])
        n98 = Index Array(array=w215) -> (element=w211:u32)  [unwired: 1 in]
        n99 = Delete From Array(array=w213, index=w211) -> (array with subset deleted=w212:T4)  [unwired: 1 in, 1 out]
        n100 = property on="Property Node" class="XYGraph (strict)"(reference=w214, error in=w209, "CrsrList"=w212) -> (error out=w208:errorcluster)  [unwired: 1 out]
      }
      event "AutoMapper": Mouse Up {
        n101 = event-data() -> ("CtlRef"=w226:refnum<vi>, "PlatMods"=w225:T22)  [unwired: 1 in, 6 out]
        n102 = property class="XYGraph (strict)"(reference=w226) -> (reference out=w218:refnum<vi>, "ActPaletteTool"=w224:i32)  [unwired: 1 in, 1 out]
        n103 = Unbundle By Name(w225) -> ("Ctrl"=w221:bool)
        n104 = Equal?(x=w224, y=2) -> (x = y?=w222:bool)
        n105 = And(x=w222, y=w221) -> (x .and. y?=w220:bool)
        n106 = And(x="Zoom\ndelete", y=w220) -> (x .and. y?=w219:bool)
        "Delete zoom" <- w219
        n107 = case shown="True" w219 {
          tunnel: w218 -> [_ w227]
          frame False {
          }
          frame True {
            n108 = property class="XYGraph (strict)"(reference=w227) -> ("XScale.Maximum"=w228:dbl, "XScale.Minimum"=w229:dbl, "YScale.Maximum"=w230:dbl, "YScale.Minimum"=w231:dbl)  [unwired: 1 in, 2 out]
            n109 = Bundle("XScale.Maximum"=w228, "XScale.Minimum"=w229, "YScale.Maximum"=w230, "YScale.Minimum"=w231) -> (→"Range":T10)  [unwired: 1 in]
          }
        }
      }
      event "Clear Cursors": Value Change {
        n110 = event-data() -> ()  [unwired: 1 in, 6 out]
        n111 = property on="Property Node" class="XYGraph (strict)"(reference=w234, "CrsrList"=T4 [] ("Cursor List")) -> ()  [unwired: 1 in, 2 out]
      }
      event "Save Cursors": Value Change {
        n112 = event-data() -> ()  [unwired: 1 in, 6 out]
        n113 = property on="Property Node" class="XYGraph (strict)"(reference=w237) -> (error out=w236:errorcluster, "CrsrList"=w235:T4)  [unwired: 1 in, 1 out]
        n114 = call "Save Cursors.vi"("Cursor List"=w235) -> ()  [unwired: 9 in, 2 out]
      }
      event "Load Cursors": Value Change {
        n115 = event-data() -> ()  [unwired: 1 in, 6 out]
        n116 = call "Get All Contacts.vi"() -> ("Cursor List"=w238:T23)  [unwired: 9 in, 2 out]
        n117 = property on="Property Node" class="XYGraph (strict)"(reference=w240, "CrsrList"=w238) -> (error out=w239:errorcluster)  [unwired: 1 in, 1 out]
      }
    }
  }
  n118 = while {
    tunnel: w4 -> [w242]
    stop <- w244 stop-if-true
    n119 = local read "output array"() -> (w241:T5)
    n120 = Wait (ms)(milliseconds to wait="Display wait") -> ()  [unwired: 1 out]
    n121 = for {
      tunnel: w241 -> [w255] mode=indexing
      shift-right: [w253] -> w245
      shift-left: cluster{cluster{"X":dbl, "Z":dbl}[]}[] [] -> [w252]
      tunnel: w242 -> [w250]
      i -> [w247]
      n122 = Unbundle By Name(w255) -> ("Line array"=w256:cluster{"X":dbl, "Y":dbl, "Z":dbl}[])
      n123 = Format Into String(format string="L%d", w247) -> (resulting string=w248:string)  [unwired: 2 in, 1 out]
      n124 = property on="Property Node" class="XYGraph (strict)"(reference=w250, "Active Plot"=w247, "Plot.Plot Name"=w248) -> (error out=→"error out 3":errorcluster)  [unwired: 1 in, 1 out]
      n125 = for {
        tunnel: w256 -> [w261] mode=indexing
        tunnel: [w258] -> w257 mode=indexing
        n126 = Unbundle By Name(w261) -> ("X"=w260:dbl, "Z"=w259:dbl)
        n127 = Bundle("X"=w260, "Z"=w259) -> (w258:cluster{"X":dbl, "Z":dbl})  [unwired: 1 in]
      }
      n128 = Bundle(w257) -> (w254:cluster{cluster{"X":dbl, "Z":dbl}[]})  [unwired: 1 in]
      n129 = Build Array (concatenate)(w252, w254) -> (w253:cluster{cluster{"X":dbl, "Z":dbl}[]}[])
    }
    "AutoMapper" <- w245
    n130 = local read "stop"() -> (w244:bool)
  }
  n131 = disable-structure shown="Disabled" {
    frame Disabled {
      n132 = property on="Property Node" class="XYGraph (strict)" props=["YScale", "ScaleFit", "YScale", "Range", "XScale", "LooseFit", "Plot Bounds", "Transpose Array", "XScale"]() -> ()  [unwired: 7 in, 3 out]
      n133 = property on="Property Node" class="XYGraph (strict)"() -> ("CrsrList"=w263:T4, "Selected Cursors"=w262:u32[])  [unwired: 2 in, 2 out]
      n134 = Index Array(array=w262) -> (element=w264:u32)  [unwired: 1 in]
      n135 = Index Array(array=w263, index=w264) -> (element=w265:T21)
      n136 = Unbundle By Name(w265) -> ()  [unwired: 1 out]
    }
    frame Enabled {
    }
  }
  n137 = Merge Errors(w6, w3) -> (w5:errorcluster)
  n138 = flat-sequence {
    tunnel: w5 -> [w266]
    frame #0 {
      "error out 4" <- w266
    }
    frame #1 {
      n139 = control-ref of="This VI"() -> (w267:refnum<vi>)
      n140 = invoke class="VI" method="FP.Close"(reference=w267) -> ()  [unwired: 2 in, 3 out]
    }
  }
